vi "Send Update Seq.vi"(7 "Message Priority (Normal)":T2=enum."Normal", 8 "error in (no error)":errorcluster, 9 "Sequence":T1(array[cluster])=[{"Duration"=0, "Value"=1, "Name"="Step1"}, {"Duration"=10, "Value"=2, "Name"="Step2"}, {"Duration"=10, "Value"=4, "Name"="Step3"}, {"Duration"=20, "Value"=0, "Name"="Step4"}, {"Duration"=20, "Value"=0, "Name"="Step5"}, {"Duration"=30, "Value"=0, "Name"="Step6"}, {"Duration"=30, "Value"=0, "Name"="Step7"}, {"Duration"=40, "Value"=0, "Name"="Step8"}, {"Duration"=40, "Value"=100, "Name"="Step9"}, {"Duration"=50, "Value"=0, "Name"="Step10"}], 10 "file path":path, 11 "Message Enqueuer":refnum<class "Message Enqueuer.lvclass">) -> (0 "error out":errorcluster, 3 "Message Enqueuer out":refnum<class "Message Enqueuer.lvclass">)   [LabVIEW 2019, in "Sequence.lvlib" / "Update Seq Msg.lvclass"]
doc: "This VI sends the message to an actor."
uses:
  Update Seq Msg.lvclass
  <vilib>/ActorFramework/Message Enqueuer/Message Enqueuer.lvclass
  <vilib>/ActorFramework/Message Enqueuer/Message Priority.ctl
  C:/Program Files (x86)/National Instruments/LabVIEW 2019/vi.lib/ActorFramework/Message/Message.lvclass
  Update Seq Msg.lvclass/Update Seq Msg.ctl
  <vilib>/ActorFramework/Message Enqueuer/Message Enqueuer.lvclass/Message Enqueuer.ctl
  <vilib>/ActorFramework/Message Priority Queue/Priority Enqueue.vi
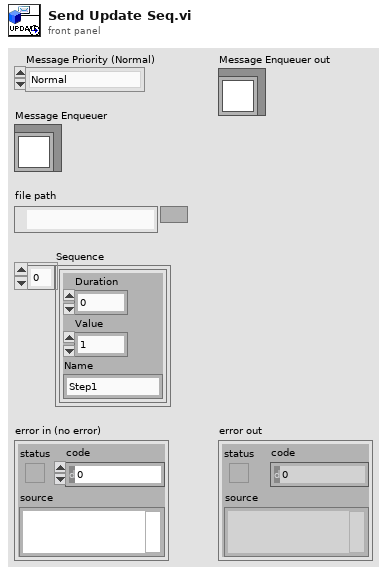
[diagram p1: front panel]
types:
  T1 = cluster{"Duration":i32, "Value":u32, "Name":string}[]
  T2 = typedef "Actor Framework.lvlib/Message Enqueuer.lvclass/Message Priority.ctl" = enum16{"Low", "Normal", "High"}
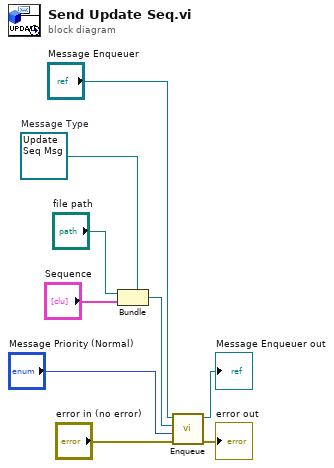
[diagram p0: block diagram]
diagram:
  w6 = refnum<class "Update Seq Msg.lvclass"> refnum  # Message Type
  n1 = Bundle(cluster=w6, "file path", "Sequence") -> (w5:refnum<class "Update Seq Msg.lvclass">)
  n2 = call <vilib>:"Enqueue.vi"("error in (no error)"="error in (no error)", "Message Priority (Normal)"="Message Priority (Normal)", "Message"=w5, "Message Enqueuer in"="Message Enqueuer") -> ("error out"=→"error out":errorcluster, "Message Enqueuer out"=→"Message Enqueuer out":refnum<class "Message Enqueuer.lvclass">)  [unwired: 6 in]
